vi "Compute (f,g)(X,Y) Arrays.vi"(8 "Error In":errorcluster, 9 "Formulas":string[](array[string]), 10 "Y Array":dbl[](array[numeric]), 11 "X Array":dbl[](array[numeric])) -> (0 "Error Out":errorcluster, 1 "Formula String":string, 2 "g(X,Y) Array":dbl[](array[numeric]), 3 "f(X,Y) Array":dbl[](array[numeric]))   [LabVIEW 2019, in "XY Graph Add-Ons.lvlib"]
uses:
  XY Graph Add-Ons.lvlib
  <vilib>/gmath/NI_Gmath.lvlib
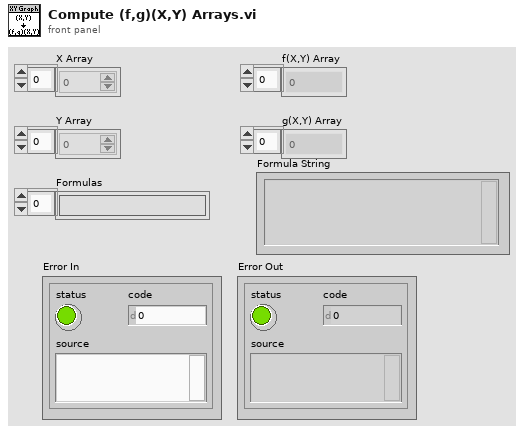
[diagram p1: front panel]
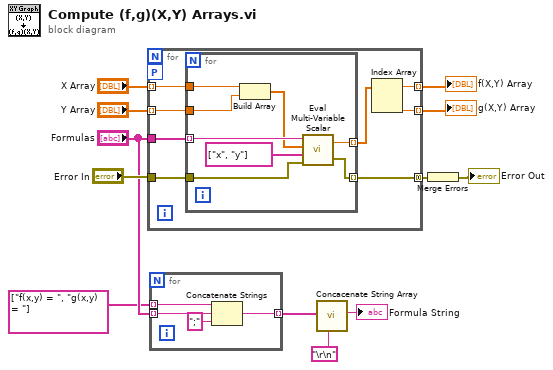
[diagram p0: block diagram]
diagram:
  n1 = for {
    tunnel: "X Array" -> [w19] mode=indexing
    tunnel: "Y Array" -> [w18] mode=indexing
    tunnel: [w14] -> w11 mode=indexing
    tunnel: [w13] -> w12 mode=indexing
    tunnel: "Formulas" -> [w20]
    tunnel: "Error In" -> [w17]
    workers-P: _ -> [_]
    tunnel: [w16] -> w7 mode=concatenating
    n2 = for {
      tunnel: w20 -> [w28] mode=indexing
      tunnel: w19 -> [w26]
      tunnel: w18 -> [w25]
      tunnel: w17 -> [w23]
      tunnel: [w22] -> w16 mode=indexing
      tunnel: [w21] -> w15 mode=indexing
      n3 = Build Array(w26, w25) -> (w24:dbl[])
      n4 = call <vilib>:"Eval Multi-Variable Scalar.vi"("error in (no error)"=w23, "Variables"=string[] ["x", "y"], "X Values"=w24, "formula"=w28) -> ("error out"=w22:errorcluster, "y value"=w21:dbl)
    }
    n5 = Index Array(array=w15) -> (element #1=w14:dbl, element #2=w13:dbl)  [unwired: 2 in]
  }
  "g(X,Y) Array" <- w12
  "f(X,Y) Array" <- w11
  n6 = for {
    tunnel: "Formulas" -> [w31] mode=indexing
    tunnel: string[] ["f(x,y) = ", "g(x,y) = "] -> [w32] mode=indexing
    tunnel: [w29] -> w3 mode=indexing
    n7 = Concatenate Strings(w32, w31, ";" ("string")) -> (w29:string)
  }
  n8 = call "Concacenate String Array.vi"("Separator (TAB)"="\r\n", "String Array"=w3) -> ("Formatted String"=→"Formula String":string)  [unwired: 9 in]
  n9 = Merge Errors(w7) -> (→"Error Out":errorcluster)
